vi "ReadQueueMessage_Cluster.vi"(6 "timeout in ms (-1)":i32=-1, 7 "preview? (F)":bool, 8 "error in":errorcluster, 11 "message ref in":refnum<class "CLM_LocalMessage_Queue.lvclass">) -> (0 "error out":errorcluster, 2 "message":T1, 3 "message ref out":refnum<class "CLM_LocalMessage_Queue.lvclass">, 4 "timed out?":bool)   [LabVIEW 2013, in "CLM_LocalMessage_Queue.lvclass"]
uses:
  CLM_LocalMessage_Queue.lvclass
  LocalMessage/Message.ctl
  CLM_LocalMessage_Queue.lvclass/CLM_LocalMessage_Queue.ctl
  LocalMessage/CLM_LocalMessage.lvclass
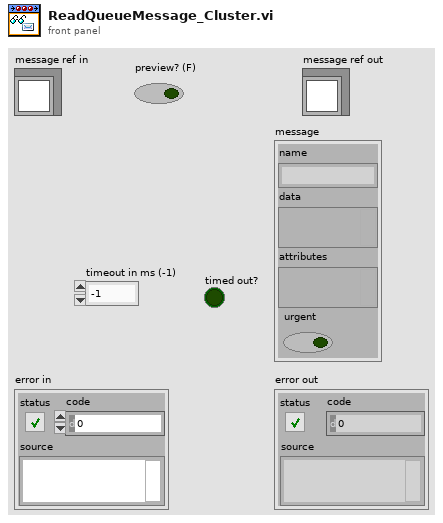
[diagram p1: front panel]
types:
  T1 = typedef "CLM_LocalMessage.lvclass/Message.ctl" = cluster{"name":string, "data":variant, "attributes":variant, "urgent":bool}
  T2 = typedef "CLM_LocalMessage_Queue.lvclass/MessageQueue.ctl" = refnum<queue>
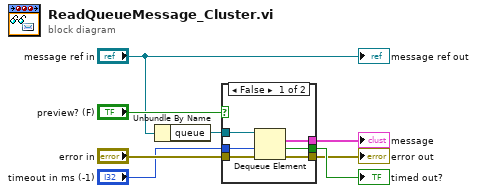
[diagram p0: block diagram]
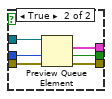
[diagram p2: hidden frame]
diagram:
  n1 = Unbundle By Name("message ref in") -> ("queue"=w1:T2)
  n2 = case shown="False" "preview? (F)" {
    tunnel: w1 -> [w14 w20]
    tunnel: "error in" -> [w13 w19]
    tunnel: "timeout in ms (-1)" -> [w12 w18]
    tunnel: [w11 w16] -> w6
    tunnel: [w10 w17] -> w5
    tunnel: [w9 w15] -> w4
    frame False {
      n3 = Dequeue Element(queue=w14, timeout in ms (-1)=w12, error in (no error)=w13) -> (element=w9:T1, timed out?=w11:bool, error out=w10:errorcluster)  [unwired: 1 out]
    }
    frame True {
      n4 = Preview Queue Element(queue=w20, timeout in ms (-1)=w18, error in (no error)=w19) -> (element=w15:T1, timed out?=w16:bool, error out=w17:errorcluster)  [unwired: 1 out]
    }
  }
  "error out" <- w5
  "timed out?" <- w6
  "message" <- w4
  "message ref out" <- "message ref in"
